vi "SENS_SWE_POIN.vi"(0 "VISA IN":refnum<visa-resource-name>, 1 "Sweep Points":i32=1, 5 "error in":errorcluster, 7 "Channel":i32=1) -> (14 "VISA Out":refnum<visa-resource-name>, 19 "error out":errorcluster)   [LabVIEW 2018, in "PNA-X.lvlib"]
doc: "SENSe<cnum>:SWEep:POINts <num> \n(Read-Write) Sets the number of data points for the measurement. \nParameters \n<cnum> Any existing channel number. If unspecified, value is set to 1 \n<num> Choose any number between 1 and 16001 \nNote: This command will accept MIN or MAX instead of a numeric parameter. See SCPI \nSyntax for more information. \nExamples SENS:SWE:POIN 51 \nsense2:sweep:points max \nQuery Syntax SENSe<cnum>:SWEep:POINts? \nReturn Type Numeric \nDefault 201"
uses:
  PNA-X.lvlib
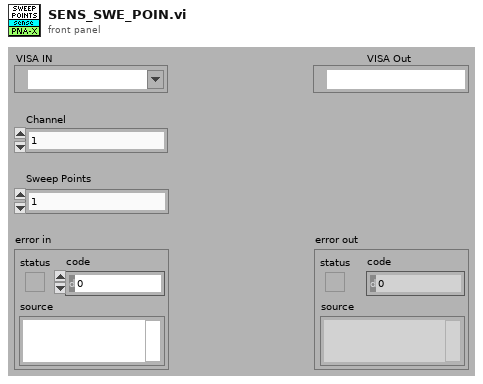
[diagram p1: front panel]
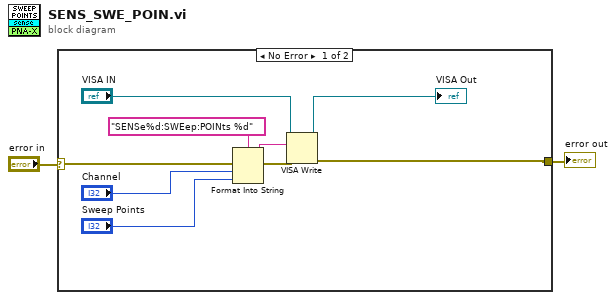
[diagram p0: block diagram]
diagram:
  n1 = case shown="No Error" "error in" {
    selector: "error in" -> [w11 w12]
    tunnel: [w6 w12] -> w1
    frame No Error {
      n2 = Format Into String(format string="SENSe%d:SWEep:POINts %d" ("Cmdline"), error in=w11, "Channel", "Sweep Points") -> (resulting string=w9:string, error out=w10:errorcluster)  [unwired: 1 in]
      n3 = VISA Write(VISA resource name="VISA IN", write buffer=w9, error in (no error)=w10) -> (VISA resource name out=→"VISA Out":refnum<visa-resource-name>, error out=w6:errorcluster)  [unwired: 1 out]
    }
    frame Error {
    }
  }
  "error out" <- w1
